vi "StringToArray.vi"(1 "spreadsheet string":string) -> (0 "array":string[](array[string]))   [LabVIEW 2010]
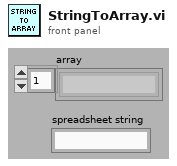
[diagram p1: front panel]
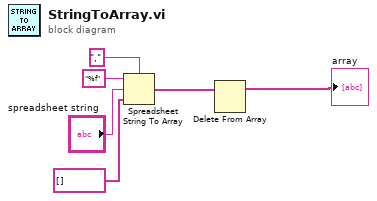
[diagram p0: block diagram]
diagram:
  n1 = Spreadsheet String To Array(delimiter (Tab)=",", format string="%f", spreadsheet string="spreadsheet string", array type (2D Dbl)=string[] [] ("Array")) -> (array=w2:string[])
  n2 = Delete From Array(array=w2) -> (array with subset deleted=→"array":string[])  [unwired: 2 in, 1 out]
